vi "set_helioscan_icon.vi"(8 "error in (no error)":errorcluster, 11 "reference cluster in":T1) -> (0 "error out":errorcluster)   [LabVIEW 2010]
uses:
  type_definitions/clusters/controls_refs.ctl
  user32.dll
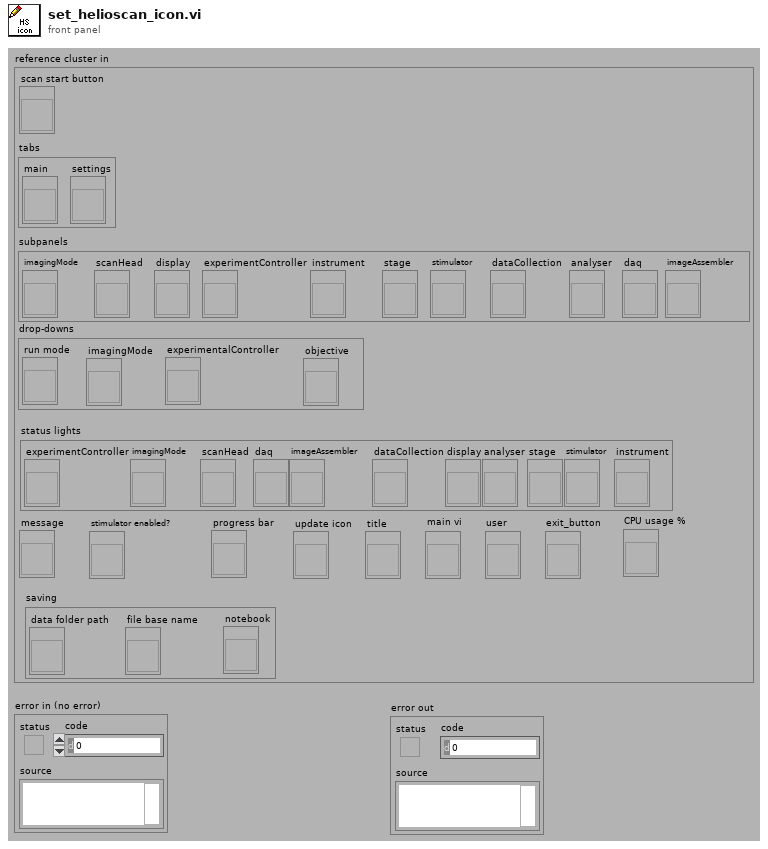
[diagram p1: front panel]
types:
  T1 = typedef "controls_refs.ctl" = cluster{"scan start button":refnum<vi>, "tabs":cluster{"main":refnum<vi>, "settings":refnum<vi>}, "subpanels":cluster{"imagingMode":refnum<vi>, "scanHead":refnum<vi>, "display":refnum<vi>, "experimentController":refnum<vi>, "instrument":refnum<vi>, "stage":refnum<vi>, "stimulator":refnum<vi>, "dataCollection":refnum<vi>, "analyser":refnum<vi>, "daq":refnum<vi>, "imageAssembler":refnum<vi>}, "drop-downs":cluster{"run mode":refnum<vi>, "imagingMode":refnum<vi>, "experimentalController":refnum<vi>, "objective":refnum<vi>}, "status lights":cluster{"experimentController":refnum<vi>, "imagingMode":refnum<vi>, "scanHead":refnum<vi>, "daq":refnum<vi>, "imageAssembler":refnum<vi>, "dataCollection":refnum<vi>, "display":refnum<vi>, "analyser":refnum<vi>, "stage":refnum<vi>, "stimulator":refnum<vi>, "instrument":refnum<vi>}, "message":refnum<vi>, "stimulator enabled?":refnum<vi>, "saving":cluster{"data folder path":refnum<vi>, "file base name":refnum<vi>, "notebook":refnum<vi>}, "progress bar":refnum<vi>, "update icon":refnum<vi>, "title":refnum<vi>, "main vi":refnum<vi>, "user":refnum<vi>, "exit_button":refnum<vi>, "CPU usage %":refnum<vi>}
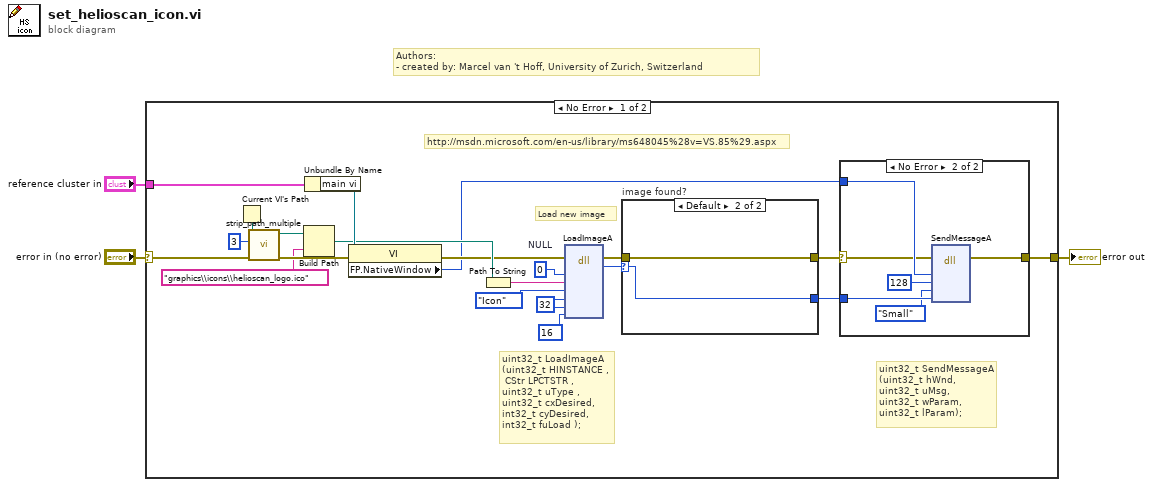
[diagram p0: block diagram]
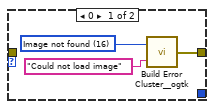
[diagram p2: hidden frame]
diagram:
  # "Authors: \n- created by: Marcel van 't Hoff, University of Zurich, Switzerland"
  n1 = case shown="No Error" "error in (no error)" {
    selector: "error in (no error)" -> [w23 w37]
    tunnel: "reference cluster in" -> [w24 _]
    tunnel: [w22 w37] -> w1
    frame No Error {
      w7 = u32 32 ("cxDesired")
      w8 = u32 0  # NULL
      # "http://msdn.microsoft.com/en-us/library/ms648045%28v=VS.85%29.aspx"
      # "uint32_t SendMessageA\n(uint32_t hWnd,\nuint32_t uMsg,\nuint32_t wParam,\nuint32_t lParam);"
      # "uint32_t LoadImageA\n(uint32_t HINSTANCE ,\n CStr LPCTSTR ,\nuint32_t uType , \nuint32_t cxDesired, \nint32_t cyDesired, \nint32_t fuLoad );"
      # "Load new image"
      n2 = Current VI's Path() -> (path=w20:path)
      n3 = call "strip_path_multiple.vi"("error in (no error)"=w23, "number of strips"=3, "path in"=w20) -> ("error out"=w19:errorcluster, "path out"=w16:path)  [unwired: 7 in]
      n4 = Build Path(base path=w16, name or relative path="graphics\\icons\\helioscan_logo.ico") -> (appended path=w15:path)
      n5 = Unbundle By Name(w24) -> ("main vi"=w21:refnum<vi>)
      n6 = property class="VI"(reference=w21, error in=w19) -> (error out=w14:errorcluster, "FP.NativeWindow"=w13:u64)  [unwired: 1 out]
      n7 = Path To String(path=w15) -> (string=w5:string)
      n8 = dll-call lib="user32.dll" fn="LoadImageA" label="LoadImage"(error in=w14, "HINSTANCE"=w8, "LPCTSTR"=w5, "uType"=enum32{"Bitmap", "Icon", "Cursor"}."Icon", "cxDesired"=w7, "cyDesired"=w7, "fuLoad"=16) -> (error out=w9:errorcluster, "ImageHandle"=w10:u32)  [unwired: 8 in, 1 out]
      n9 = case "image found?" shown="Default" w10 {
        selector: w10 -> [_ w28]
        tunnel: [_ w28] -> w11
        tunnel: [w25 w29] -> w12
        tunnel: w9 -> [_ w29]
        frame 0 {
          w27 = 16 items=["No error", "Argument error", "Memory is full", "Out of zone", "End of file", "File already open", "Generic file I/O error", "File not found", "File permission error", "Disk is full", "Duplicate path", "Too many files open", "System feature not enabled", "Resource file not found", "Cannot add resource", "Resource not found", "Image not found", "Image memory error", "Pen does not exist", "Config type invalid", "Config token not found", "Config parse error", "Config memory error", "Bad external code format", "Bad external code offset", "External code not present", "Null window", "Destroy window error", "Null menu", "Print aborted", "Bad print record", "Print driver error", "Windows error during printing", "Memory error during printing", "Print dialog error", "Generic print error", "Invalid device refnum", "Device not found", "Device parameter error", "Device unit error", "Cannot open device", "Device call aborted", "Generic error", "Cancelled by user", "Object ID too low", "Object ID too high", "Object not in heap", "Unknown heap", "Unknown object (invalid DefProc)", "Unknown object (DefProc not in table)", "Message out of range", "Invalid (null) method", "Unknown message", "Manager call not supported", "Bad address", "Network operation in progress", "Network operation timed out", "Connection is busy", "Network attribute not supported", "Network error", "Address in use", "System out of memory", "Connection aborted", "Connection refused", "Not connected", "Already connected", "Connection closed", "Initialization error (interapplication manager)", "Bad occurrence", "Wait on unbound occurrence handler", "Occurrence queue overflow", "Datalog type conflict", "Unused", "Unrecognized type (interapplication manager)", "Memory corrupt", "Failed to make temporary DLL", "Old CIN version", "Drag socket not found", "Failed to load drop-object", "Failed to register OLE object", "Failed to release OLE object", "Format specifier type mismatch", "Unknown format specifier", "Too few format specifiers", "Too many format specifiers", "Scan failed", "Newer CIN version", "Error converting to variant", "Runtime menu error", "Password tampered", "Variant attribute not found", "Incompatible variant data type", "Event data is not available", "Event Store is not present", "Occurrence is not found", "Event Queue is not created", "Event info is not available", "Refnum passed is NULL", "Error retrieving Class GUID", "Error retrieving CoClass GUID", "Error retrieving TypeLib GUID.", "Bad built application magic bytes.", "Specific driver is different from the specific driver associated with the Logical Name.", "There is no session opened to the class driver.", "Max Error", "MAX - Error with config objects", "MAX - Error loading configuration", "MAX - Group not supported"]
          n10 = call <userlib>:"Build Error Cluster__ogtk.vi"("String to Prepend to source (\"\")"="Could not load image" ("source"), "code"=w27) -> ("error out"=w25:errorcluster)
        }
        frame Default {
        }
      }
      n11 = case shown="No Error" w12 {
        selector: w12 -> [w30 w33]
        tunnel: [w30 w36] -> w22
        tunnel: w13 -> [_ w35]
        tunnel: w11 -> [_ w34]
        frame Error {
        }
        frame No Error {
          n12 = dll-call lib="user32.dll" fn="SendMessageA" label="SendMessage"(error in=w33, "hWnd"=w35, "uMsg"=u32 128 ("dimension size"), "wParam"=enum32{"Small", "Big"}."Small", "lParam"=w34) -> (error out=w36:errorcluster)  [unwired: 7 in, 1 out]
        }
      }
    }
    frame Error {
    }
  }
  "error out" <- w1
